vi "startHWError.vi"(8 "error in (no error)":errorcluster, 11 "AtomChipHWC in":refnum<class "AtomChipHWC.lvclass">) -> (0 "error out":errorcluster, 2 "error":bool, 3 "AtomChipHWC out":refnum<class "AtomChipHWC.lvclass">)   [LabVIEW 2011, in "Hardware.lvlib" / "HWControllers.lvlib" / "AtomChipHWC.lvclass"]
uses:
  AtomChipHWC.lvclass
  AtomChipHWC.lvclass/AtomChipHWC.ctl
  Channels/Digital/DigitalOutput.lvclass
  Channels/VoltOutput/AnalogOutput.lvclass
  Channels/DDSOutput/Generic/DDSOutput.lvclass
  HWController.lvclass
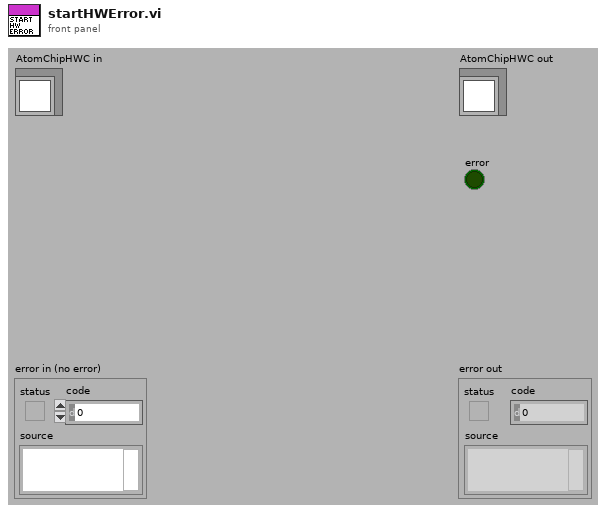
[diagram p1: front panel]
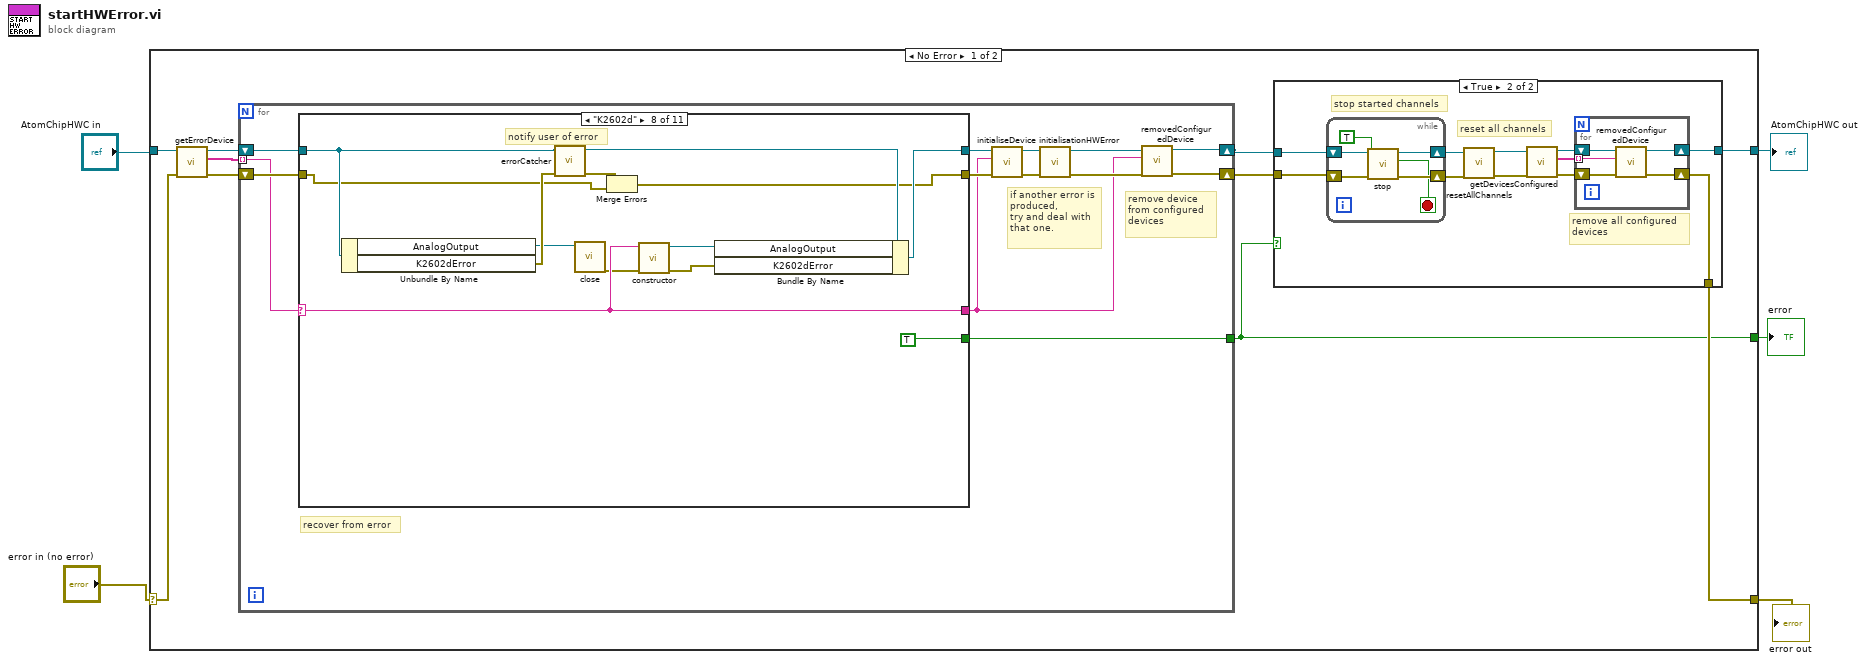
[diagram p0: block diagram]
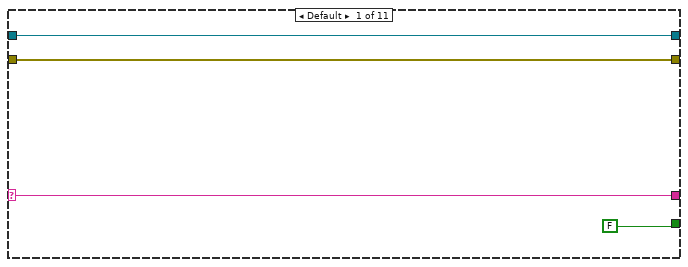
[diagram p3: hidden frame]
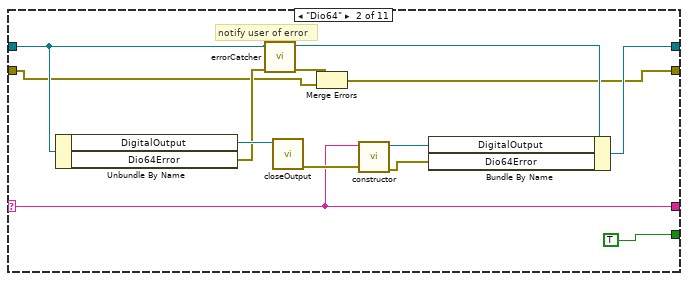
[diagram p4: hidden frame]
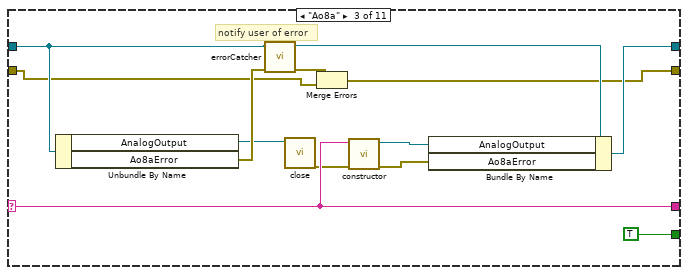
[diagram p5: hidden frame]
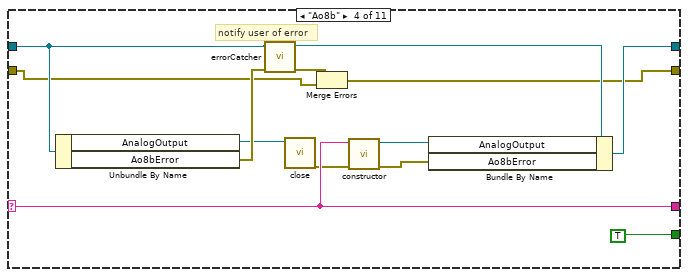
[diagram p6: hidden frame]
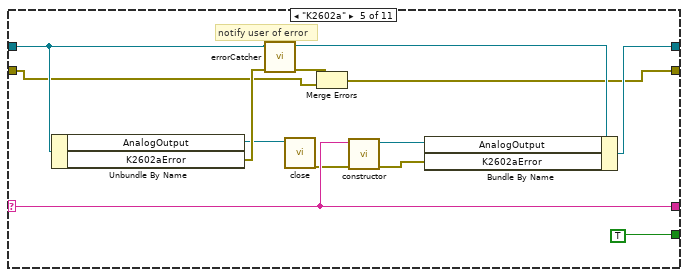
[diagram p7: hidden frame]
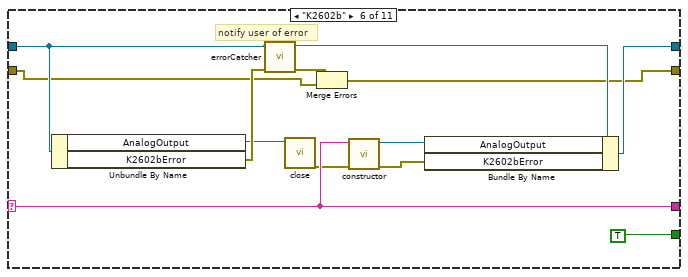
[diagram p8: hidden frame]
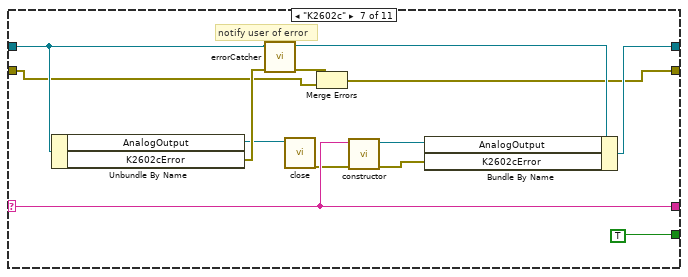
[diagram p9: hidden frame]
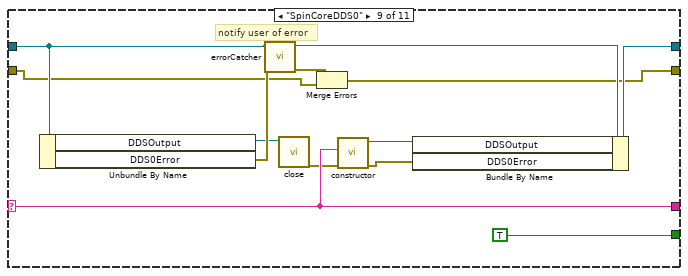
[diagram p10: hidden frame]
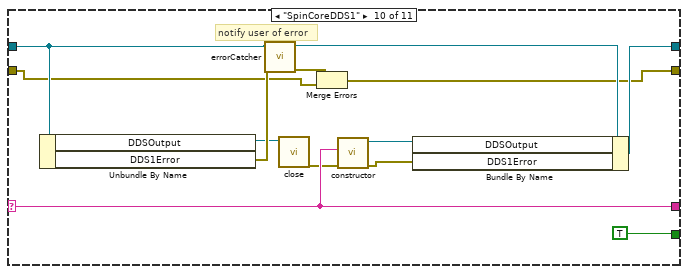
[diagram p11: hidden frame]
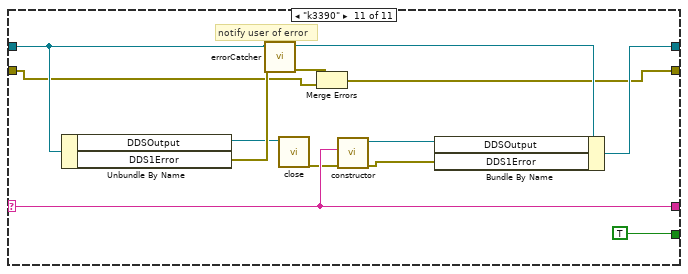
[diagram p12: hidden frame]
diagram:
  n1 = case shown="No Error" "error in (no error)" {
    selector: "error in (no error)" -> [w14 w187]
    tunnel: "AtomChipHWC in" -> [w15 w188]
    tunnel: [w9 w188] -> w2
    tunnel: [w10 w187] -> w3
    tunnel: [w6 _] -> w1
    frame No Error {
      n2 = call "getErrorDevice.vi"("error in (no error)"=w14, "AtomChipHWC in"=w15) -> ("error out"=w11:errorcluster, "Devices"=w12:string[], "AtomChipHWC out"=w13:refnum<class "AtomChipHWC.lvclass">)  [unwired: 7 in]
      n3 = for {
        tunnel: w12 -> [w50] mode=indexing
        shift-right: [w44] -> w8
        shift-left: w13 -> [w52]
        shift-right: [w43] -> w7
        shift-left: w11 -> [w51]
        tunnel: [w40] -> w6
        # "remove device\nfrom configured\ndevices"
        # "if another error is\nproduced,\ntry and deal with\nthat one."
        # "recover from error"
        n4 = case shown="\"K2602d\"" w50 {
          selector: w50 -> [w54 w58 w74 w87 w100 w113 w126 w139 w150 w163 w176]
          tunnel: w52 -> [w56 w65 w82 w95 w108 w121 w134 w147 w160 w173 w186]
          tunnel: [w56 w60 w77 w90 w103 w116 w129 w142 w155 w168 w181] -> w45
          tunnel: [w55 w59 w76 w89 w102 w115 w128 w141 w154 w167 w180] -> w42
          tunnel: w51 -> [w55 w61 w78 w91 w104 w117 w130 w143 w156 w169 w182]
          tunnel: [w54 w58 w74 w87 w100 w113 w126 w139 w150 w163 w176] -> w41
          tunnel: [FALSE TRUE TRUE TRUE TRUE TRUE TRUE TRUE TRUE TRUE TRUE] -> w40
          frame Default {
          }
          frame "Dio64" {
            # "notify user of error"
            n5 = Unbundle By Name(w65) -> ("DigitalOutput"=w69:refnum<class "DigitalOutput.lvclass">, "Dio64Error"=w63:errorcluster)
            n6 = call-dynamic "errorCatcher.vi"("error in (no error)"=w63, "HWController in"=w65) -> ("error out"=w62:errorcluster, "HWController out"=w64:refnum<class "AtomChipHWC.lvclass">)  [unwired: 8 in]
            n7 = call-dynamic "closeOutput.vi"("DigitalOutput in"=w69) -> ("error out"=w68:errorcluster)  [unwired: 10 in]
            n8 = Merge Errors(w62, w61) -> (w59:errorcluster)
            n9 = call "constructor.vi"("error in (no error)"=w68, "deviceName"=w58) -> ("error out"=w66:errorcluster, "DigitalOutput out"=w67:refnum<class "DigitalOutput.lvclass">)  [unwired: 8 in]
            n10 = Bundle By Name(cluster=w64, "DigitalOutput"=w67, "Dio64Error"=w66) -> (w60:refnum<class "AtomChipHWC.lvclass">)
          }
          frame "Ao8a" {
            # "notify user of error"
            n11 = Unbundle By Name(w82) -> ("AnalogOutput"=w75:refnum<class "AnalogOutput.lvclass">, "Ao8aError"=w80:errorcluster)
            n12 = call-dynamic "errorCatcher.vi"("error in (no error)"=w80, "HWController in"=w82) -> ("error out"=w79:errorcluster, "HWController out"=w81:refnum<class "AtomChipHWC.lvclass">)  [unwired: 8 in]
            n13 = call-dynamic "close.vi"("AnalogOutput in"=w75) -> ("error out"=w73:errorcluster)  [unwired: 10 in]
            n14 = Merge Errors(w79, w78) -> (w76:errorcluster)
            n15 = call "constructor.vi"("error in (no error)"=w73, "deviceName"=w74) -> ("error out"=w71:errorcluster, "AnalogOutput out"=w72:refnum<class "AnalogOutput.lvclass">)  [unwired: 8 in]
            n16 = Bundle By Name(cluster=w81, "AnalogOutput"=w72, "Ao8aError"=w71) -> (w77:refnum<class "AtomChipHWC.lvclass">)
          }
          frame "Ao8b" {
            # "notify user of error"
            n17 = Unbundle By Name(w95) -> ("AnalogOutput"=w88:refnum<class "AnalogOutput.lvclass">, "Ao8bError"=w93:errorcluster)
            n18 = call-dynamic "errorCatcher.vi"("error in (no error)"=w93, "HWController in"=w95) -> ("error out"=w92:errorcluster, "HWController out"=w94:refnum<class "AtomChipHWC.lvclass">)  [unwired: 8 in]
            n19 = call-dynamic "close.vi"("AnalogOutput in"=w88) -> ("error out"=w86:errorcluster)  [unwired: 10 in]
            n20 = Merge Errors(w92, w91) -> (w89:errorcluster)
            n21 = call "constructor.vi"("error in (no error)"=w86, "deviceName"=w87) -> ("error out"=w84:errorcluster, "AnalogOutput out"=w85:refnum<class "AnalogOutput.lvclass">)  [unwired: 8 in]
            n22 = Bundle By Name(cluster=w94, "AnalogOutput"=w85, "Ao8bError"=w84) -> (w90:refnum<class "AtomChipHWC.lvclass">)
          }
          frame "K2602a" {
            # "notify user of error"
            n23 = Unbundle By Name(w108) -> ("AnalogOutput"=w101:refnum<class "AnalogOutput.lvclass">, "K2602aError"=w106:errorcluster)
            n24 = call-dynamic "errorCatcher.vi"("error in (no error)"=w106, "HWController in"=w108) -> ("error out"=w105:errorcluster, "HWController out"=w107:refnum<class "AtomChipHWC.lvclass">)  [unwired: 8 in]
            n25 = call-dynamic "close.vi"("AnalogOutput in"=w101) -> ("error out"=w99:errorcluster)  [unwired: 10 in]
            n26 = Merge Errors(w105, w104) -> (w102:errorcluster)
            n27 = call "constructor.vi"("error in (no error)"=w99, "deviceName"=w100) -> ("error out"=w97:errorcluster, "AnalogOutput out"=w98:refnum<class "AnalogOutput.lvclass">)  [unwired: 8 in]
            n28 = Bundle By Name(cluster=w107, "AnalogOutput"=w98, "K2602aError"=w97) -> (w103:refnum<class "AtomChipHWC.lvclass">)
          }
          frame "K2602b" {
            # "notify user of error"
            n29 = Unbundle By Name(w121) -> ("AnalogOutput"=w114:refnum<class "AnalogOutput.lvclass">, "K2602bError"=w119:errorcluster)
            n30 = call-dynamic "errorCatcher.vi"("error in (no error)"=w119, "HWController in"=w121) -> ("error out"=w118:errorcluster, "HWController out"=w120:refnum<class "AtomChipHWC.lvclass">)  [unwired: 8 in]
            n31 = call-dynamic "close.vi"("AnalogOutput in"=w114) -> ("error out"=w112:errorcluster)  [unwired: 10 in]
            n32 = Merge Errors(w118, w117) -> (w115:errorcluster)
            n33 = call "constructor.vi"("error in (no error)"=w112, "deviceName"=w113) -> ("error out"=w110:errorcluster, "AnalogOutput out"=w111:refnum<class "AnalogOutput.lvclass">)  [unwired: 8 in]
            n34 = Bundle By Name(cluster=w120, "AnalogOutput"=w111, "K2602bError"=w110) -> (w116:refnum<class "AtomChipHWC.lvclass">)
          }
          frame "K2602c" {
            # "notify user of error"
            n35 = Unbundle By Name(w134) -> ("AnalogOutput"=w127:refnum<class "AnalogOutput.lvclass">, "K2602cError"=w132:errorcluster)
            n36 = call-dynamic "errorCatcher.vi"("error in (no error)"=w132, "HWController in"=w134) -> ("error out"=w131:errorcluster, "HWController out"=w133:refnum<class "AtomChipHWC.lvclass">)  [unwired: 8 in]
            n37 = call-dynamic "close.vi"("AnalogOutput in"=w127) -> ("error out"=w125:errorcluster)  [unwired: 10 in]
            n38 = Merge Errors(w131, w130) -> (w128:errorcluster)
            n39 = call "constructor.vi"("error in (no error)"=w125, "deviceName"=w126) -> ("error out"=w123:errorcluster, "AnalogOutput out"=w124:refnum<class "AnalogOutput.lvclass">)  [unwired: 8 in]
            n40 = Bundle By Name(cluster=w133, "AnalogOutput"=w124, "K2602cError"=w123) -> (w129:refnum<class "AtomChipHWC.lvclass">)
          }
          frame "K2602d" {
            # "notify user of error"
            n41 = Unbundle By Name(w147) -> ("AnalogOutput"=w140:refnum<class "AnalogOutput.lvclass">, "K2602dError"=w145:errorcluster)
            n42 = call-dynamic "errorCatcher.vi"("error in (no error)"=w145, "HWController in"=w147) -> ("error out"=w144:errorcluster, "HWController out"=w146:refnum<class "AtomChipHWC.lvclass">)  [unwired: 8 in]
            n43 = call-dynamic "close.vi"("AnalogOutput in"=w140) -> ("error out"=w138:errorcluster)  [unwired: 10 in]
            n44 = Merge Errors(w144, w143) -> (w141:errorcluster)
            n45 = call "constructor.vi"("error in (no error)"=w138, "deviceName"=w139) -> ("error out"=w136:errorcluster, "AnalogOutput out"=w137:refnum<class "AnalogOutput.lvclass">)  [unwired: 8 in]
            n46 = Bundle By Name(cluster=w146, "AnalogOutput"=w137, "K2602dError"=w136) -> (w142:refnum<class "AtomChipHWC.lvclass">)
          }
          frame "SpinCoreDDS0" {
            # "notify user of error"
            n47 = Unbundle By Name(w160) -> ("DDSOutput"=w153:refnum<class "DDSOutput.lvclass">, "DDS0Error"=w158:errorcluster)
            n48 = call-dynamic "errorCatcher.vi"("error in (no error)"=w158, "HWController in"=w160) -> ("error out"=w157:errorcluster, "HWController out"=w159:refnum<class "AtomChipHWC.lvclass">)  [unwired: 8 in]
            n49 = call-dynamic "close.vi"("DDSOutput in"=w153) -> ("error out"=w149:errorcluster)  [unwired: 10 in]
            n50 = Merge Errors(w157, w156) -> (w154:errorcluster)
            n51 = call "constructor.vi"("error in (no error)"=w149, "device"=w150) -> ("error out"=w151:errorcluster, "DDSOutput out"=w152:refnum<class "DDSOutput.lvclass">)  [unwired: 8 in]
            n52 = Bundle By Name(cluster=w159, "DDSOutput"=w152, "DDS0Error"=w151) -> (w155:refnum<class "AtomChipHWC.lvclass">)
          }
          frame "SpinCoreDDS1" {
            # "notify user of error"
            n53 = Unbundle By Name(w173) -> ("DDSOutput"=w166:refnum<class "DDSOutput.lvclass">, "DDS1Error"=w171:errorcluster)
            n54 = call-dynamic "errorCatcher.vi"("error in (no error)"=w171, "HWController in"=w173) -> ("error out"=w170:errorcluster, "HWController out"=w172:refnum<class "AtomChipHWC.lvclass">)  [unwired: 8 in]
            n55 = call-dynamic "close.vi"("DDSOutput in"=w166) -> ("error out"=w162:errorcluster)  [unwired: 10 in]
            n56 = Merge Errors(w170, w169) -> (w167:errorcluster)
            n57 = call "constructor.vi"("error in (no error)"=w162, "device"=w163) -> ("error out"=w164:errorcluster, "DDSOutput out"=w165:refnum<class "DDSOutput.lvclass">)  [unwired: 8 in]
            n58 = Bundle By Name(cluster=w172, "DDSOutput"=w165, "DDS1Error"=w164) -> (w168:refnum<class "AtomChipHWC.lvclass">)
          }
          frame "k3390" {
            # "notify user of error"
            n59 = Unbundle By Name(w186) -> ("DDSOutput"=w179:refnum<class "DDSOutput.lvclass">, "DDS1Error"=w184:errorcluster)
            n60 = call-dynamic "errorCatcher.vi"("error in (no error)"=w184, "HWController in"=w186) -> ("error out"=w183:errorcluster, "HWController out"=w185:refnum<class "AtomChipHWC.lvclass">)  [unwired: 8 in]
            n61 = call-dynamic "close.vi"("DDSOutput in"=w179) -> ("error out"=w175:errorcluster)  [unwired: 10 in]
            n62 = Merge Errors(w183, w182) -> (w180:errorcluster)
            n63 = call "constructor.vi"("error in (no error)"=w175, "device"=w176) -> ("error out"=w177:errorcluster, "DDSOutput out"=w178:refnum<class "DDSOutput.lvclass">)  [unwired: 8 in]
            n64 = Bundle By Name(cluster=w185, "DDSOutput"=w178, "DDS1Error"=w177) -> (w181:refnum<class "AtomChipHWC.lvclass">)
          }
        }
        n65 = call "initialiseDevice.vi"("error in (no error)"=w42, "deviceName"=w41, "AtomChipHWC in"=w45) -> ("error out"=w48:errorcluster, "AtomChipHWC out"=w49:refnum<class "AtomChipHWC.lvclass">)  [unwired: 7 in]
        n66 = call-dynamic "initialisationHWError.vi"("error in (no error)"=w48, "AtomChipHWC in"=w49) -> ("error out"=w46:errorcluster, "AtomChipHWC out"=w47:refnum<class "AtomChipHWC.lvclass">)  [unwired: 8 in]
        n67 = call-dynamic "removedConfiguredDevice.vi"("error in (no error)"=w46, "device"=w41, "HWController in"=w47) -> ("error out"=w43:errorcluster, "HWController out"=w44:refnum<class "AtomChipHWC.lvclass">)  [unwired: 7 in]
      }
      n68 = case shown="True" w6 {
        tunnel: [w16 w24] -> w10
        tunnel: [w17 w23] -> w9
        tunnel: w8 -> [w17 w21]
        tunnel: w7 -> [w16 w20]
        frame False {
          # "no error"
        }
        frame True {
          # "stop started channels"
          # "remove all configured\ndevices"
          # "reset all channels"
          n69 = while {
            shift-right: [w32] -> w19
            shift-left: w21 -> [w34]
            shift-right: [w31] -> w18
            shift-left: w20 -> [w33]
            stop <- w30 stop-if-true
            n70 = call-dynamic "stop.vi"("error in (no error)"=w33, "stop?"=TRUE, "AtomChipHWC in"=w34) -> ("error out"=w31:errorcluster, "stopped"=w30:bool, "AtomChipHWC out"=w32:refnum<class "AtomChipHWC.lvclass">)  [unwired: 6 in]
          }
          n71 = call-dynamic "resetAllChannels.vi"("error in (no error)"=w18, "AtomChipHWC in"=w19) -> ("error out"=w27:errorcluster, "AtomChipHWC out"=w28:refnum<class "AtomChipHWC.lvclass">)  [unwired: 8 in]
          n72 = call "getDevicesConfigured.vi"("error in (no error)"=w27, "HWController.lvclass in"=w28) -> ("error out"=w25:errorcluster, "devicesConfigured"=w22:string[], "HWController.lvclass out"=w26:refnum<class "AtomChipHWC.lvclass">)  [unwired: 7 in]
          n73 = for {
            shift-right: [w38] -> w23
            shift-left: w26 -> [w39]
            shift-right: [w36] -> w24
            shift-left: w25 -> [w37]
            tunnel: w22 -> [w35] mode=indexing
            n74 = call-dynamic "removedConfiguredDevice.vi"("error in (no error)"=w37, "device"=w35, "HWController in"=w39) -> ("error out"=w36:errorcluster, "HWController out"=w38:refnum<class "AtomChipHWC.lvclass">)  [unwired: 7 in]
          }
        }
      }
    }
    frame Error {
    }
  }
  "error out" <- w3
  "AtomChipHWC out" <- w2
  "error" <- w1
